vi "refresh.vi"(8 "error in (no error)":errorcluster, 10 "Engine Configuration In":refnum<class "engine configuration.lvclass">, 11 "TDMS datalogger editor node In":refnum<class "TDMS datalogger editor node.lvclass">) -> (0 "error out":errorcluster, 2 "Engine Configuration Out":refnum<class "engine configuration.lvclass">, 3 "TDMS datalogger editor node Out":refnum<class "TDMS datalogger editor node.lvclass">)   [LabVIEW 2013, in "TDMS datalogger editor node.lvclass"]
uses:
  TDMS datalogger editor node.lvclass
  <vilib>/NI/Module Execution Interface/Engine Configuration/engine configuration.lvclass
  TDMS datalogger editor node.lvclass/TDMS datalogger editor node.ctl
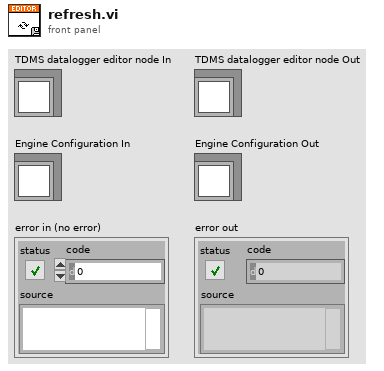
[diagram p1: front panel]
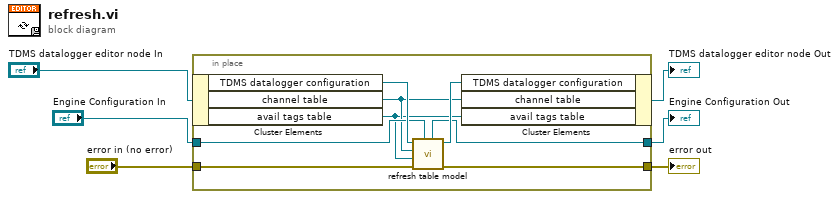
[diagram p0: block diagram]
diagram:
  n1 = in-place {
    in-place-border: "Engine Configuration In" -> [w12]
    in-place-border: [w11] -> w4
    in-place-border: "error in (no error)" -> [w10]
    in-place-border: [w9] -> w2
    n2 = in-place-cluster #1("TDMS datalogger editor node In") -> ("TDMS datalogger configuration"=w14:refnum<class "TDMS datalogger configuration.lvclass">, "channel table"=w8:refnum<vi>, "avail tags table"=w7:refnum<vi>)
    n3 = call "refresh table model.vi"("engine configuration"=w12, "error in"=w10, "avail tags"=w7, "chan table"=w8, "TDMS datalogger configuration"=w14) -> ("error out"=w9:errorcluster, "TDMS datalogger configuration out"=w13:refnum<class "TDMS datalogger configuration.lvclass">, "engine configuration out"=w11:refnum<class "engine configuration.lvclass">)  [unwired: 4 in]
    n4 = in-place-cluster #1("TDMS datalogger configuration"=w13, "channel table"=w8, "avail tags table"=w7) -> (→"TDMS datalogger editor node Out":refnum<class "TDMS datalogger editor node.lvclass">)
  }
  "Engine Configuration Out" <- w4
  "error out" <- w2
